vi "Get Function.vi"(8 "error in (no error)":errorcluster caption="entrée d'erreur (pas d'erreur)", 11 "Class Multimeter (Default) en entrée":refnum<class "Class Multimeter (Default).lvclass">) -> (0 "error out":errorcluster caption="sortie d'erreur", 2 "Function":T1, 3 "Class Multimeter (Default) en sortie":refnum<class "Class Multimeter (Default).lvclass">)   [LabVIEW 2020, in "Library Instrument & Equipement.lvlib" / "Library Multimeter.lvlib" / "Class Multimeter (Default).lvclass"]
uses:
  Class Multimeter (Default).lvclass
  Commun VI/TypeDef/Command Multimeter/Typedef Function.ctl
  Class Multimeter (Default).lvclass/Class Multimeter (Default).ctl
  Commun VI/Library Commun.lvlib
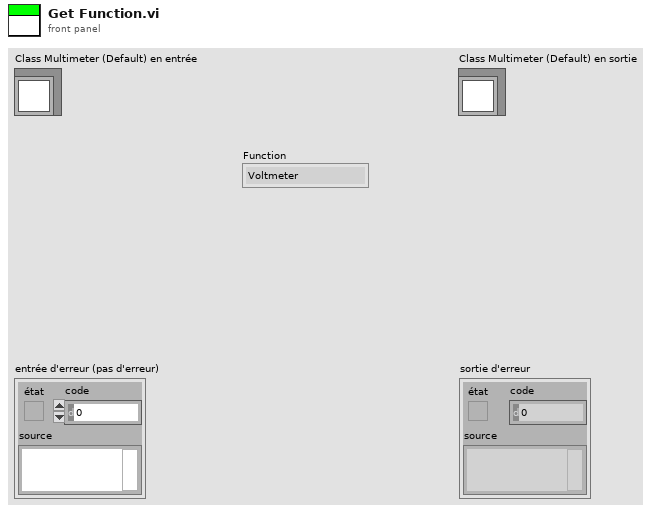
[diagram p1: front panel]
types:
  T1 = typedef "Library Commun.lvlib/Typedef Function.ctl" = enum16{"Voltmeter", "Ammeter", "Continuity", "Ohmmeter", "Frequencymeter"}
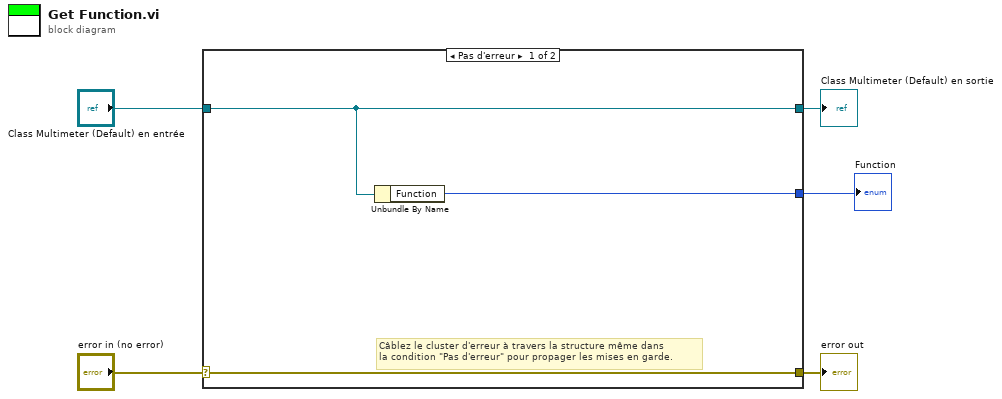
[diagram p0: block diagram]
diagram:
  n1 = case shown="Pas d'erreur" "error in (no error)" {
    selector: "error in (no error)" -> [w8 w10]
    tunnel: [w8 w10] -> w4
    tunnel: [w7 w9] -> w2
    tunnel: "Class Multimeter (Default) en entrée" -> [w7 w9]
    tunnel: [w6 _] -> w1
    frame No Error {
      # "Câblez le cluster d'erreur à travers la structure même dans\nla condition \"Pas d'erreur\" pour propager les mises en garde."
      n2 = Unbundle By Name(w7) -> ("Function"=w6:T1)
    }
    frame Error {
    }
  }
  "error out" <- w4
  "Class Multimeter (Default) en sortie" <- w2
  "Function" <- w1
